vi "Do.vi"(8 "error in (no error)":errorcluster, 10 "Actor in":refnum<class "Actor.lvclass">, 11 "Ensure Cell is Off Msg":refnum<class "Set Cell Value.lvclass">) -> (0 "error out":errorcluster, 2 "Actor out":refnum<class "Actor.lvclass">)   [LabVIEW 2021, in "Grid Screen.lvlib" / "Set Cell Value.lvclass"]
doc: "This VI delivers the message to the actor by calling the appropriate method(s) on the actor."
uses:
  Set Cell Value.lvclass
  <vilib>/ActorFramework/Actor/Actor.lvclass
  Set Cell Value.lvclass/Set Cell Value.ctl
  MC Screen/Grid Screen.lvclass
  C:/Program Files/National Instruments/LabVIEW 2024/vi.lib/ActorFramework/Actor/Actor.lvclass
  9ef47adc-f318-494c-9b8b-6df3216d6863.vi
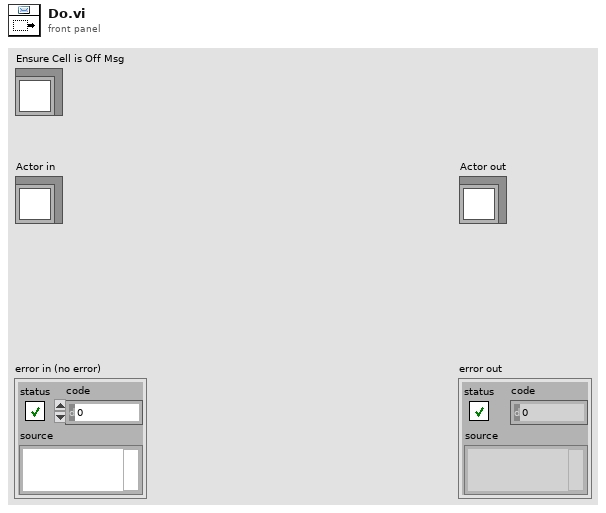
[diagram p1: front panel]
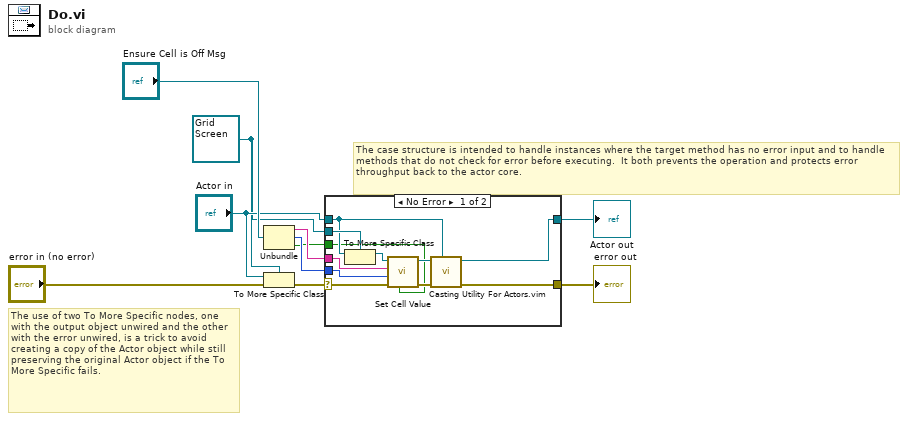
[diagram p0: block diagram]
diagram:
  w4 = refnum<class "Grid Screen.lvclass"> refnum ("Actor in")
  # "The use of two To More Specific nodes, one with the output object unwired and the other with the error unwired, is a trick to avoid creating a copy of the Actor object while still preserving the original Actor object if the To More Specific fails."
  # "The case structure is intended to handle instances where the target method has no error input and to handle methods that do not check for error before executing.  It both prevents the operation and protects error throughput back to the actor core."
  n1 = Unbundle("Ensure Cell is Off Msg") -> (w3:string, w2:u32, w1:bool)
  n2 = To More Specific Class(target class=w4, reference="Actor in", error in="error in (no error)") -> (error out=w8:errorcluster)  [unwired: 1 out]
  n3 = case shown="No Error" w8 {
    selector: w8 -> [w21 w23]
    tunnel: [w15 w23] -> w7
    tunnel: [w16 w22] -> w6
    tunnel: "Actor in" -> [w18 w22]
    tunnel: w4 -> [w19 _]
    tunnel: w3 -> [w13 _]
    tunnel: w2 -> [w12 _]
    tunnel: w1 -> [w11 _]
    frame No Error {
      n4 = To More Specific Class(target class=w19, reference=w18) -> (specific class reference=w20:refnum<class "Grid Screen.lvclass">)  [unwired: 1 in, 1 out]
      n5 = call-dynamic "Set Cell Value.vi"("Value"=w11, "error in (no error)"=w21, "Difficulty"=w12, "Category"=w13, "Grid Screen in"=w20) -> ("error out"=w14:errorcluster, "Grid Screen out"=w17:refnum<class "Grid Screen.lvclass">)  [unwired: 5 in]
      n6 = call "Casting Utility For Actors.vim"("type"=w18, "error in (no error)"=w14, "Actor in"=w17) -> ("error out"=w15:errorcluster, "Actor out"=w16:refnum<class "Actor.lvclass">)  [unwired: 7 in]
    }
    frame Error {
      # "If type check fails, pass the original object out again."
    }
  }
  "error out" <- w7
  "Actor out" <- w6
